vi "Get Strength of a Hand.vi"(0 "Cards in a hand":string[](array[string]), 1 "F:J is Normal Card | T:J is Joker Card (F)":bool) -> (2 "Strength of a Hand":i32[](array[numeric]))   [LabVIEW 2020, in "AoC 2023.lvlib"]
uses:
  AoC 2023.lvlib
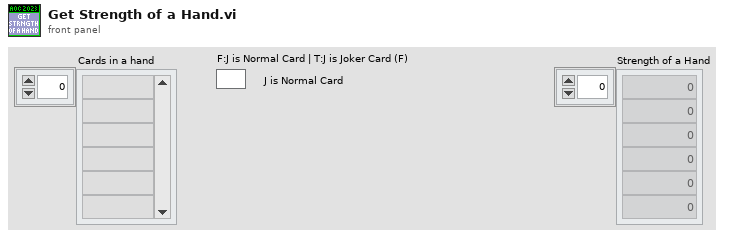
[diagram p1: front panel]
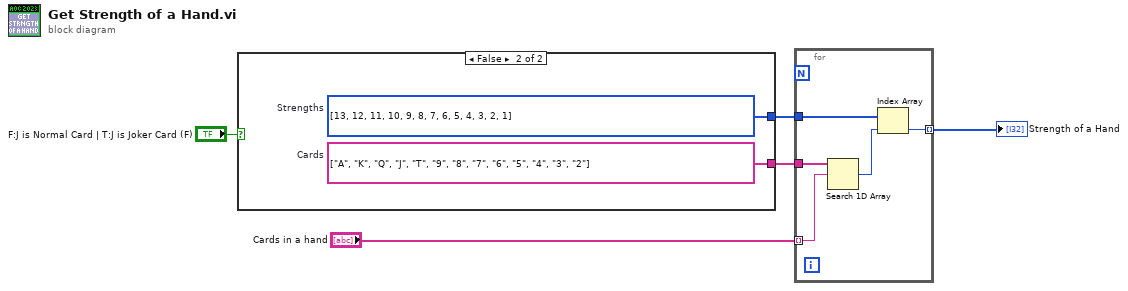
[diagram p0: block diagram]
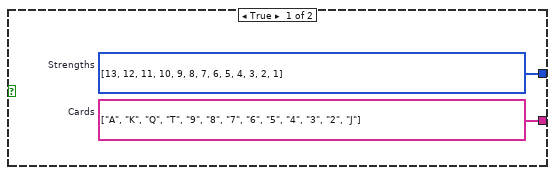
[diagram p2: hidden frame]
diagram:
  n1 = case shown="False" "F:J is Normal Card | T:J is Joker Card (F)" {
    tunnel: [w7 w9] -> w5
    tunnel: [w6 w8] -> w4
    frame True {
      w6 = i32[] [13, 12, 11, 10, 9, 8, 7, 6, 5, 4, 3, 2, 1]  # Strengths
      w7 = string[] ["A", "K", "Q", "T", "9", "8", "7", "6", "5", "4", "3", "2", "J"]  # Cards
    }
    frame False {
      w8 = i32[] [13, 12, 11, 10, 9, 8, 7, 6, 5, 4, 3, 2, 1]  # Strengths
      w9 = string[] ["A", "K", "Q", "J", "T", "9", "8", "7", "6", "5", "4", "3", "2"]  # Cards
    }
  }
  n2 = for {
    tunnel: w5 -> [w14]
    tunnel: w4 -> [w13]
    tunnel: "Cards in a hand" -> [w11] mode=indexing
    tunnel: [w10] -> w2 mode=indexing
    n3 = Search 1D Array(1D array=w14, element=w11) -> (index of element=w12:i32)  [unwired: 1 in]
    n4 = Index Array(array=w13, index=w12) -> (element=w10:i32)
  }
  "Strength of a Hand" <- w2
